vi "Read Config.vi"(8 "error in":errorcluster, 11 "file path":path=path "C:/Project/20-020_W601/trunk/config.ini") -> (0 "error out":errorcluster, 1 "Password":string, 2 "output cluster":T1={"LH"={"Go Up"={"Min Speed"=120.0, "Max Speed"=10.0, "Min Time"=1.82, "Max Time"=3.7, "Min Run Current"=0.0, "Max Run Current"=10.0, "Min Stall Current"=0.0, "Max Stall Current"=25.0, "Min Stall Force"=170.0, "Max Stall Force"=320.0, "Min Stroke"=170.0, "Max Stroke"=320.0}, "Go Down"={"Min Speed"=10.0, "Max Speed"=250.0, "Min Travel Time"=1.82, "Max Travel Time"=3.7, "Min Run Current"=0.0, "Max Run Current"=10.0}, "Shipping"={"Min Distance"=150.0, "Max Distance"=300.0, "Setpoint"=5.0}, "Anti-Pinch"={"Min Force"=5.0, "Max Force"=15.0}}, "RH"={"Go Up"={"Min Speed"=120.0, "Max Speed"=10.0, "Min Time"=1.82, "Max Time"=3.7, "Min Run Current"=0.0, "Max Run Current"=10.0, "Min Stall Current"=0.0, "Max Stall Current"=25.0, "Min Stall Force"=170.0, "Max Stall Force"=320.0, "Min Stroke"=170.0, "Max Stroke"=320.0}, "Go Down"={"Min Speed"=10.0, "Max Speed"=250.0, "Min Travel Time"=1.82, "Max Travel Time"=3.7, "Min Run Current"=0.0, "Max Run Current"=10.0}, "Shipping"={"Min Distance"=150.0, "Max Distance"=300.0, "Setpoint"=5.0}, "Anti-Pinch"={"Min Force"=5.0, "Max Force"=15.0}}, "W 601 FR RH Std"={"Go Up"={"Min Speed"=10.0, "Max Speed"=250.0, "Min Time"=0.5, "Max Time"=4.3, "Min Run Current"=0.0, "Max Run Current"=10.0, "Min Stall Current"=0.0, "Max Stall Current"=25.0, "Min Stall Force"=170.0, "Max Stall Force"=320.0, "Min Stroke"=254.4, "Max Stroke"=270.4}, "Go Down"={"Min Speed"=10.0, "Max Speed"=250.0, "Min Travel Time"=0.5, "Max Travel Time"=4.3, "Min Run Current"=0.0, "Max Run Current"=10.0}, "Shipping"={"Min Distance"=5.0, "Max Distance"=15.0, "Setpoint"=5.0}, "Anti-Pinch"={"Min Force"=5.0, "Max Force"=15.0}}, "W 601 FR LH Std"={"Go Up"={"Min Speed"=10.0, "Max Speed"=250.0, "Min Time"=0.5, "Max Time"=4.3, "Min Run Current"=0.0, "Max Run Current"=10.0, "Min Stall Current"=0.0, "Max Stall Current"=25.0, "Min Stall Force"=170.0, "Max Stall Force"=320.0, "Min Stroke"=254.4, "Max Stroke"=270.4}, "Go Down"={"Min Speed"=10.0, "Max Speed"=250.0, "Min Travel Time"=0.5, "Max Travel Time"=4.3, "Min Run Current"=0.0, "Max Run Current"=10.0}, "Shipping"={"Min Distance"=5.0, "Max Distance"=15.0, "Setpoint"=5.0}, "Anti-Pinch"={"Min Force"=5.0, "Max Force"=15.0}}, "W 601 RR RH Std"={"Go Up"={"Min Speed"=10.0, "Max Speed"=250.0, "Min Time"=0.5, "Max Time"=4.3, "Min Run Current"=0.0, "Max Run Current"=10.0, "Min Stall Current"=0.0, "Max Stall Current"=25.0, "Min Stall Force"=170.0, "Max Stall Force"=320.0, "Min Stroke"=254.4, "Max Stroke"=270.4}, "Go Down"={"Min Speed"=10.0, "Max Speed"=250.0, "Min Travel Time"=0.5, "Max Travel Time"=4.3, "Min Run Current"=0.0, "Max Run Current"=10.0}, "Shipping"={"Min Distance"=5.0, "Max Distance"=15.0, "Setpoint"=5.0}, "Anti-Pinch"={"Min Force"=5.0, "Max Force"=15.0}}, "W 601 RR LH Std"={"Go Up"={"Min Speed"=10.0, "Max Speed"=250.0, "Min Time"=0.5, "Max Time"=4.3, "Min Run Current"=0.0, "Max Run Current"=10.0, "Min Stall Current"=0.0, "Max Stall Current"=25.0, "Min Stall Force"=170.0, "Max Stall Force"=320.0, "Min Stroke"=254.4, "Max Stroke"=270.4}, "Go Down"={"Min Speed"=10.0, "Max Speed"=250.0, "Min Travel Time"=0.5, "Max Travel Time"=4.3, "Min Run Current"=0.0, "Max Run Current"=10.0}, "Shipping"={"Min Distance"=5.0, "Max Distance"=15.0, "Setpoint"=5.0}, "Anti-Pinch"={"Min Force"=5.0, "Max Force"=15.0}}, "W 601 FR RH AP"={"Go Up"={"Min Speed"=10.0, "Max Speed"=250.0, "Min Time"=0.5, "Max Time"=4.3, "Min Run Current"=0.0, "Max Run Current"=10.0, "Min Stall Current"=0.0, "Max Stall Current"=25.0, "Min Stall Force"=170.0, "Max Stall Force"=320.0, "Min Stroke"=254.4, "Max Stroke"=270.4}, "Go Down"={"Min Speed"=10.0, "Max Speed"=250.0, "Min Travel Time"=0.5, "Max Travel Time"=4.3, "Min Run Current"=0.0, "Max Run Current"=10.0}, "Shipping"={"Min Distance"=5.0, "Max Distance"=15.0, "Setpoint"=5.0}, "Anti-Pinch"={"Min Force"=5.0, "Max Force"=15.0}}, "W 601 FR LH AP"={"Go Up"={"Min Speed"=10.0, "Max Speed"=250.0, "Min Time"=0.5, "Max Time"=4.3, "Min Run Current"=0.0, "Max Run Current"=10.0, "Min Stall Current"=0.0, "Max Stall Current"=25.0, "Min Stall Force"=170.0, "Max Stall Force"=320.0, "Min Stroke"=254.4, "Max Stroke"=270.4}, "Go Down"={"Min Speed"=10.0, "Max Speed"=250.0, "Min Travel Time"=0.5, "Max Travel Time"=4.3, "Min Run Current"=0.0, "Max Run Current"=10.0}, "Shipping"={"Min Distance"=5.0, "Max Distance"=15.0, "Setpoint"=5.0}, "Anti-Pinch"={"Min Force"=5.0, "Max Force"=15.0}}, "W 601 RR RH AP"={"Go Up"={"Min Speed"=10.0, "Max Speed"=250.0, "Min Time"=0.5, "Max Time"=4.3, "Min Run Current"=0.0, "Max Run Current"=10.0, "Min Stall Current"=0.0, "Max Stall Current"=25.0, "Min Stall Force"=170.0, "Max Stall Force"=320.0, "Min Stroke"=254.4, "Max Stroke"=270.4}, "Go Down"={"Min Speed"=10.0, "Max Speed"=250.0, "Min Travel Time"=0.5, "Max Travel Time"=4.3, "Min Run Current"=0.0, "Max Run Current"=10.0}, "Shipping"={"Min Distance"=5.0, "Max Distance"=15.0, "Setpoint"=5.0}, "Anti-Pinch"={"Min Force"=5.0, "Max Force"=15.0}}, "W 601 RR LH AP"={"Go Up"={"Min Speed"=10.0, "Max Speed"=250.0, "Min Time"=0.5, "Max Time"=4.3, "Min Run Current"=0.0, "Max Run Current"=10.0, "Min Stall Current"=0.0, "Max Stall Current"=25.0, "Min Stall Force"=170.0, "Max Stall Force"=320.0, "Min Stroke"=254.4, "Max Stroke"=270.4}, "Go Down"={"Min Speed"=10.0, "Max Speed"=250.0, "Min Travel Time"=0.5, "Max Travel Time"=4.3, "Min Run Current"=0.0, "Max Run Current"=10.0}, "Shipping"={"Min Distance"=5.0, "Max Distance"=15.0, "Setpoint"=5.0}, "Anti-Pinch"={"Min Force"=5.0, "Max Force"=15.0}}}, 3 "file path out":path, 5 "Shipping":dbl)   [LabVIEW 2017]
doc: "v1.1:\n- Added Sense ON Delay\n\nv1.0:\nRead 2WR Motor Bencg or not."
uses:
  controls/All Specs.ctl
  controls/Specifications.ctl
  <vilib>/Utility/config.llb/Read Key (Double).vi
  <vilib>/Utility/config.llb/Read Key (String).vi
  <vilib>/Utility/config.llb/NI_LVConfig.lvlib
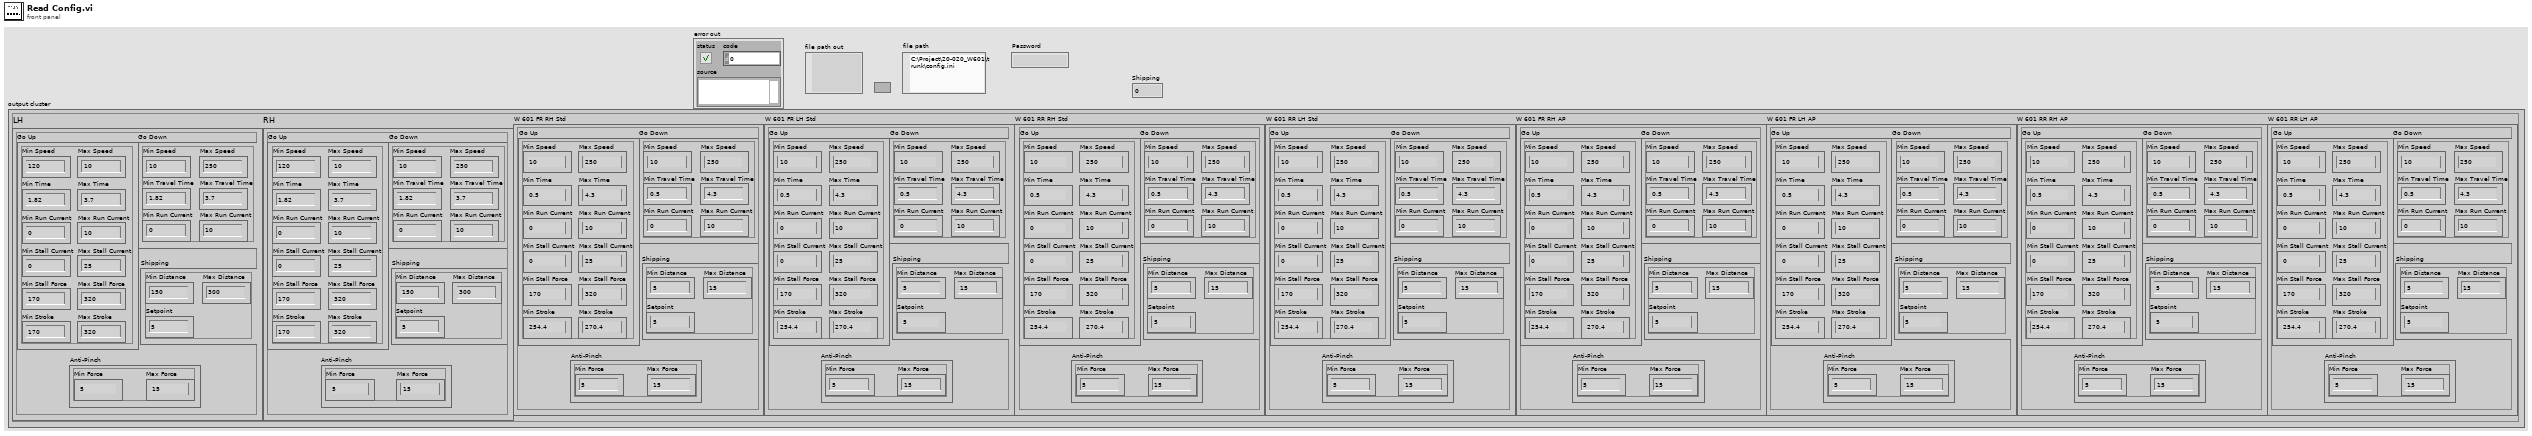
[diagram p1: front panel]
types:
  T1 = typedef "All Specs.ctl" = cluster{"LH":T2, "RH":T2, "W 601 FR RH Std":T2, "W 601 FR LH Std":T2, "W 601 RR RH Std":T2, "W 601 RR LH Std":T2, "W 601 FR RH AP":T2, "W 601 FR LH AP":T2, "W 601 RR RH AP":T2, "W 601 RR LH AP":T2}
  T2 = typedef "Specifications.ctl" = cluster{"Go Up":cluster{"Min Speed":dbl, "Max Speed":dbl, "Min Time":dbl, "Max Time":dbl, "Min Run Current":dbl, "Max Run Current":dbl, "Min Stall Current":dbl, "Max Stall Current":dbl, "Min Stall Force":dbl, "Max Stall Force":dbl, "Min Stroke":dbl, "Max Stroke":dbl}, "Go Down":cluster{"Min Speed":dbl, "Max Speed":dbl, "Min Travel Time":dbl, "Max Travel Time":dbl, "Min Run Current":dbl, "Max Run Current":dbl}, "Shipping":cluster{"Min Distance":dbl, "Max Distance":dbl, "Setpoint":dbl}, "Anti-Pinch":cluster{"Min Force":dbl, "Max Force":dbl}}
  T3 = typedef "NI_LVConfig.lvlib/Config Data RefNum.ctl" = refnum<k1>
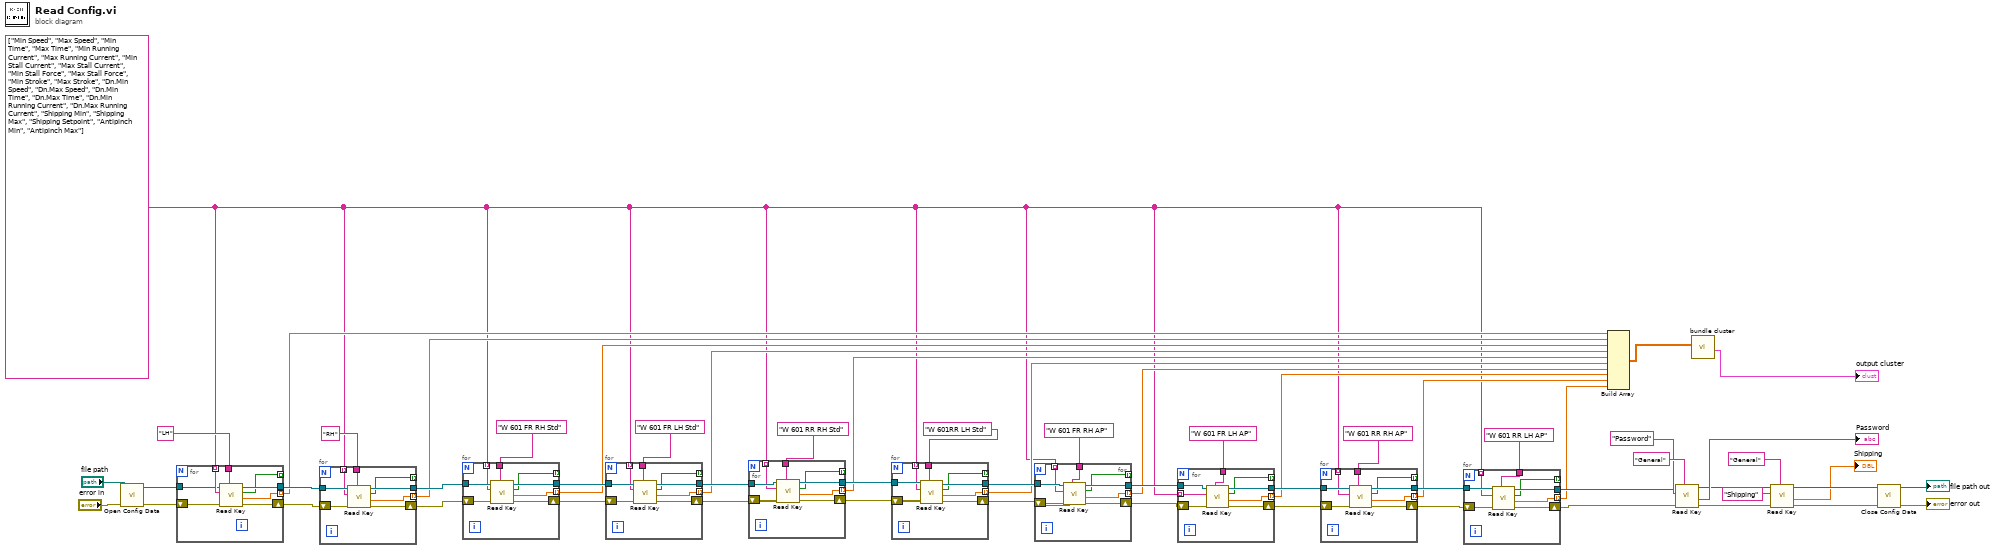
[diagram p0: block diagram]
diagram:
  w3 = string[] ["Min Speed", "Max Speed", "Min Time", "Max Time", "Min Running Current", "Max Running Current", "Min Stall Current", "Max Stall Current", "Min Stall Force", "Max Stall Force", "Min Stroke", "Max Stroke", "Dn.Min Speed", "Dn.Max Speed", "Dn.Min Time", "Dn.Max Time", "Dn.Min Running Current", "Dn.Max Running Current", "Shipping Min", "Shipping Max", "Shipping Setpoint", "Antipinch Min", "Antipinch Max"]
  n1 = call <vilib>:"Open Config Data.vi"("error in (no error)"="error in", "configuration file path"="file path") -> ("error out"=w50:errorcluster, "refnum"=w51:T3)  [unwired: 7 in, 1 out]
  n2 = for {
    tunnel: "LH" ("section") -> [w66]
    tunnel: [w65] -> w54
    shift-right: [w64] -> w55
    shift-left: w50 -> [w67]
    tunnel: [w63] -> _ mode=indexing
    tunnel: w3 -> [w62] mode=indexing
    tunnel: w51 -> [w61]
    tunnel: [w60] -> w13 mode=indexing
    n3 = call-poly <vilib>:"Read Key.vi"("section"=w66, "error in (no error)"=w67, "key"=w62, "refnum"=w61) -> ("error out"=w64:errorcluster, "value"=w60:dbl, "found?"=w63:bool, "refnum out"=w65:T3)  [unwired: 4 in]
  }
  n4 = for {
    tunnel: w54 -> [w74]
    tunnel: "RH" ("section") -> [w73]
    shift-right: [w72] -> w36
    shift-left: w55 -> [w75]
    tunnel: [w71] -> w39
    tunnel: [w70] -> _ mode=indexing
    tunnel: w3 -> [w69] mode=indexing
    tunnel: [w68] -> w12 mode=indexing
    n5 = call-poly <vilib>:"Read Key.vi"("section"=w73, "error in (no error)"=w75, "key"=w69, "refnum"=w74) -> ("error out"=w72:errorcluster, "value"=w68:dbl, "found?"=w70:bool, "refnum out"=w71:T3)  [unwired: 4 in]
  }
  n6 = for {
    shift-right: [w82] -> w37
    shift-left: w36 -> [w83]
    tunnel: [w81] -> w38
    tunnel: [w80] -> _ mode=indexing
    tunnel: [w79] -> w11 mode=indexing
    tunnel: w39 -> [w78]
    tunnel: w3 -> [w77] mode=indexing
    tunnel: "W 601 FR RH Std" -> [w76]
    n7 = call-poly <vilib>:"Read Key.vi"("section"=w76, "error in (no error)"=w83, "key"=w77, "refnum"=w78) -> ("error out"=w82:errorcluster, "value"=w79:dbl, "found?"=w80:bool, "refnum out"=w81:T3)  [unwired: 4 in]
  }
  n8 = for {
    shift-right: [w90] -> w34
    shift-left: w37 -> [w91]
    tunnel: [w89] -> w35
    tunnel: [w88] -> _ mode=indexing
    tunnel: [w87] -> w10 mode=indexing
    tunnel: w38 -> [w86]
    tunnel: w3 -> [w85] mode=indexing
    tunnel: "W 601 FR LH Std" -> [w84]
    n9 = call-poly <vilib>:"Read Key.vi"("section"=w84, "error in (no error)"=w91, "key"=w85, "refnum"=w86) -> ("error out"=w90:errorcluster, "value"=w87:dbl, "found?"=w88:bool, "refnum out"=w89:T3)  [unwired: 4 in]
  }
  n10 = for {
    shift-right: [w98] -> w32
    shift-left: w34 -> [w99]
    tunnel: [w97] -> w33
    tunnel: [w96] -> _ mode=indexing
    tunnel: [w95] -> w9 mode=indexing
    tunnel: w35 -> [w94]
    tunnel: w3 -> [w93] mode=indexing
    tunnel: "W 601 RR RH Std" -> [w92]
    n11 = call-poly <vilib>:"Read Key.vi"("section"=w92, "error in (no error)"=w99, "key"=w93, "refnum"=w94) -> ("error out"=w98:errorcluster, "value"=w95:dbl, "found?"=w96:bool, "refnum out"=w97:T3)  [unwired: 4 in]
  }
  n12 = for {
    shift-right: [w106] -> w30
    shift-left: w32 -> [w107]
    tunnel: [w105] -> w31
    tunnel: [w104] -> _ mode=indexing
    tunnel: [w103] -> w8 mode=indexing
    tunnel: w33 -> [w102]
    tunnel: w3 -> [w101] mode=indexing
    tunnel: "W 601RR LH Std" -> [w100]
    n13 = call-poly <vilib>:"Read Key.vi"("section"=w100, "error in (no error)"=w107, "key"=w101, "refnum"=w102) -> ("error out"=w106:errorcluster, "value"=w103:dbl, "found?"=w104:bool, "refnum out"=w105:T3)  [unwired: 4 in]
  }
  n14 = for {
    shift-right: [w114] -> w28
    shift-left: w30 -> [w115]
    tunnel: [w113] -> w29
    tunnel: [w112] -> _ mode=indexing
    tunnel: [w111] -> w7 mode=indexing
    tunnel: w31 -> [w110]
    tunnel: "W 601 FR RH AP" -> [w109]
    tunnel: w3 -> [w108] mode=indexing
    n15 = call-poly <vilib>:"Read Key.vi"("section"=w109, "error in (no error)"=w115, "key"=w108, "refnum"=w110) -> ("error out"=w114:errorcluster, "value"=w111:dbl, "found?"=w112:bool, "refnum out"=w113:T3)  [unwired: 4 in]
  }
  n16 = for {
    shift-right: [w122] -> w26
    shift-left: w28 -> [w123]
    tunnel: [w121] -> w27
    tunnel: [w120] -> _ mode=indexing
    tunnel: [w119] -> w6 mode=indexing
    tunnel: w29 -> [w118]
    tunnel: "W 601 FR LH AP" -> [w117]
    tunnel: w3 -> [w116] mode=indexing
    n17 = call-poly <vilib>:"Read Key.vi"("section"=w117, "error in (no error)"=w123, "key"=w116, "refnum"=w118) -> ("error out"=w122:errorcluster, "value"=w119:dbl, "found?"=w120:bool, "refnum out"=w121:T3)  [unwired: 4 in]
  }
  n18 = for {
    shift-right: [w130] -> w24
    shift-left: w26 -> [w131]
    tunnel: [w129] -> w25
    tunnel: [w128] -> _ mode=indexing
    tunnel: [w127] -> w5 mode=indexing
    tunnel: w27 -> [w125]
    tunnel: "W 601 RR RH AP" -> [w126]
    tunnel: w3 -> [w124] mode=indexing
    n19 = call-poly <vilib>:"Read Key.vi"("section"=w126, "error in (no error)"=w131, "key"=w124, "refnum"=w125) -> ("error out"=w130:errorcluster, "value"=w127:dbl, "found?"=w128:bool, "refnum out"=w129:T3)  [unwired: 4 in]
  }
  n20 = for {
    shift-right: [w138] -> w22
    shift-left: w24 -> [w139]
    tunnel: [w137] -> w23
    tunnel: [w136] -> _ mode=indexing
    tunnel: [w135] -> w4 mode=indexing
    tunnel: w25 -> [w134]
    tunnel: "W 601 RR LH AP" -> [w133]
    tunnel: w3 -> [w132] mode=indexing
    n21 = call-poly <vilib>:"Read Key.vi"("section"=w133, "error in (no error)"=w139, "key"=w132, "refnum"=w134) -> ("error out"=w138:errorcluster, "value"=w135:dbl, "found?"=w136:bool, "refnum out"=w137:T3)  [unwired: 4 in]
  }
  n22 = Build Array(w13, w12, w11, w10, w9, w8, w7, w6, w5, w4) -> (w2:dbl[][])
  n23 = call-poly <vilib>:"Read Key.vi"("section"="General", "error in (no error)"=w22, "key"="Password", "refnum"=w23) -> ("error out"=w43:errorcluster, "value"=→"Password":string, "refnum out"=w44:T3)  [unwired: 4 in, 1 out]
  n24 = call "bundle cluster.vi"("Array 3"=w2) -> ("output cluster"=→"output cluster":T1)  [unwired: 9 in]
  n25 = call-poly <vilib>:"Read Key.vi"("section"="General", "error in (no error)"=w43, "key"="Shipping", "refnum"=w44) -> ("error out"=w42:errorcluster, "value"=→"Shipping":dbl, "refnum out"=w41:T3)  [unwired: 4 in, 1 out]
  n26 = call <vilib>:"Close Config Data.vi"("error in (no error)"=w42, "refnum"=w41) -> ("error out"=→"error out":errorcluster, "file path"=→"file path out":path)  [unwired: 8 in]
